vi "UHR-Fleezers Control (host) - 10.7.vi"() -> ()   [LabVIEW 2011] (continued)
        n2234 = Build Array (concatenate)(w3488, w3486) -> (w3487:dbl[])
        n2235 = local read "Scan steps (MCL)"() -> (w3468:u64)
        n2236 = Select(t=w3581, s=w3485, f=w3563) -> (s? t:f=w3567:dbl[])
        n2237 = feedback-in #17(w3567) -> ()
        n2238 = Select(t=w3486, s=w3485, f=w3487) -> (s? t:f=w3469:dbl[])
        n2239 = feedback-in #18(w3469) -> ()
        n2240 = local read "Scan lines (y)"() -> (w3454:u64)
        n2241 = local read "N APD Samp/step"() -> (w3470:dbl)
        n2242 = feedback #19(w3512) -> (w3569:dbl[])
        n2243 = Build Array (concatenate)(w3569, w3512) -> (w3560:dbl[])
        n2244 = feedback #20(w3519) -> (w3579:dbl[])
        n2245 = Build Array (concatenate)(w3579, w3519) -> (w3578:dbl[])
        n2246 = feedback #21(w3514) -> (w3571:dbl[])
        n2247 = Build Array (concatenate)(w3571, w3514) -> (w3572:dbl[])
        n2248 = Select(t=w3512, s=w3485, f=w3560) -> (s? t:f=w3516:dbl[])
        n2249 = feedback-in #19(w3516) -> ()
        n2250 = Select(t=w3519, s=w3485, f=w3578) -> (s? t:f=w3518:dbl[])
        n2251 = feedback-in #20(w3518) -> ()
        n2252 = Select(t=w3514, s=w3485, f=w3572) -> (s? t:f=w3517:dbl[])
        n2253 = feedback-in #21(w3517) -> ()
        n2254 = Multiply(x=w3468, y=u64 2) -> (x*y=w3453:u64)
        n2255 = call "integrate 1D array interval - double.vi"("Ave N"=w3470, "Array In"=w3469) -> ("Array Out"=w3481:dbl[])  [unwired: 1 out]
        n2256 = call "integrate 1D array interval - double.vi"("Ave N"=w3470, "Array In"=w3567) -> ("Array Out"=w3566:dbl[])  [unwired: 1 out]
        n2257 = Array Size(array=w3481) -> (size(s)=w3482:i32)
        n2258 = Array Size(array=w3566) -> (size(s)=w3568:i32)
        n2259 = Multiply(x=w3454, y=w3453) -> (x*y=w3484:u64)
        n2260 = Multiply(x=w3454, y=w3453) -> (x*y=w3576:u64)
        n2261 = call <vilib>:"Mean.vi"("X"=w3516) -> ("mean"=w3500:dbl)  [unwired: 1 out]
        n2262 = Subtract(x=w3484, y=w3482) -> (x-y=w3475:u64)
        n2263 = call <vilib>:"Mean.vi"("X"=w3518) -> ("mean"=w3505:dbl)  [unwired: 1 out]
        n2264 = call <vilib>:"Mean.vi"("X"=w3517) -> ("mean"=w3503:dbl)  [unwired: 1 out]
        n2265 = call <vilib>:"Mean.vi"("X"=w3481) -> ("mean"=w3472:dbl)  [unwired: 1 out]
        n2266 = Subtract(x=w3576, y=w3568) -> (x-y=w3510:u64)
        n2267 = call <vilib>:"Mean.vi"("X"=w3566) -> ("mean"=w3507:dbl)  [unwired: 1 out]
        n2268 = Initialize Array(1.0 ("element"), w3475) -> (w3471:dbl[])
        n2269 = Initialize Array(1.0 ("element"), w3510) -> (w3501:dbl[])
        n2270 = Multiply(x=w3471, y=w3472) -> (x*y=w3473:dbl[])
        n2271 = Multiply(x=w3501, y=w3503) -> (x*y=w3504:dbl[])
        n2272 = Multiply(x=w3501, y=w3505) -> (x*y=w3506:dbl[])
        n2273 = Multiply(x=w3501, y=w3500) -> (x*y=w3502:dbl[])
        n2274 = Multiply(x=w3501, y=w3507) -> (x*y=w3508:dbl[])
        n2275 = Build Array (concatenate)(w3516, w3502) -> (w3570:dbl[])
        n2276 = Build Array (concatenate)(w3518, w3506) -> (w3574:dbl[])
        n2277 = Build Array (concatenate)(w3517, w3504) -> (w3573:dbl[])
        n2278 = Build Array (concatenate)(w3481, w3473) -> (w3483:dbl[])
        n2279 = Build Array (concatenate)(w3566, w3508) -> (w3575:dbl[])
        n2280 = Reshape Array(w3570, w3454, w3453) -> (w3536:dbl[][])
        n2281 = Reshape Array(w3483, w3454, w3453) -> (w3479:dbl[][])
        n2282 = Reshape Array(w3574, w3454, w3453) -> (w3528:dbl[][])
        n2283 = Reshape Array(w3573, w3454, w3453) -> (w3543:dbl[][])
        n2284 = Reshape Array(w3575, w3454, w3453) -> (w3553:dbl[][])
        n2285 = Array Subset(array=w3543, index (col)=0 ("index"), length (col)=w3468) -> (w3548:dbl[][])  [unwired: 2 in]
        n2286 = Array Subset(array=w3543, index (col)=w3468) -> (w3546:dbl[][])  [unwired: 3 in]
        n2287 = Array Subset(array=w3528, index (col)=0 ("index"), length (col)=w3468) -> (w3534:dbl[][])  [unwired: 2 in]
        n2288 = Array Subset(array=w3528, index (col)=w3468) -> (w3532:dbl[][])  [unwired: 3 in]
        n2289 = Array Subset(array=w3479, index (col)=0 ("index"), length (col)=w3468) -> (w3478:dbl[][])  [unwired: 2 in]
        n2290 = Array Subset(array=w3479, index (col)=w3468) -> (w3476:dbl[][])  [unwired: 3 in]
        n2291 = Array Subset(array=w3553, index (col)=0 ("index"), length (col)=w3468) -> (w3552:dbl[][])  [unwired: 2 in]
        n2292 = Array Subset(array=w3553, index (col)=w3468) -> (w3550:dbl[][])  [unwired: 3 in]
        n2293 = Array Subset(array=w3536, index (col)=0 ("index"), length (col)=w3468) -> (w3541:dbl[][])  [unwired: 2 in]
        n2294 = Array Subset(array=w3536, index (col)=w3468) -> (w3539:dbl[][])  [unwired: 3 in]
        n2295 = for {
          tunnel: w3548 -> [w3590] mode=indexing
          tunnel: [w3589] -> w3547 mode=indexing
          workers-P: _ -> [_]
          n2296 = Reverse 1D Array(array=w3590) -> (reversed array=w3589:dbl[])
        }
        n2297 = for {
          tunnel: w3534 -> [w3586] mode=indexing
          tunnel: [w3585] -> w3533 mode=indexing
          workers-P: _ -> [_]
          n2298 = Reverse 1D Array(array=w3586) -> (reversed array=w3585:dbl[])
        }
        n2299 = for {
          tunnel: w3478 -> [w3584] mode=indexing
          tunnel: [w3583] -> w3477 mode=indexing
          workers-P: _ -> [_]
          n2300 = Reverse 1D Array(array=w3584) -> (reversed array=w3583:dbl[])
        }
        n2301 = for {
          tunnel: w3552 -> [w3592] mode=indexing
          tunnel: [w3591] -> w3551 mode=indexing
          workers-P: _ -> [_]
          n2302 = Reverse 1D Array(array=w3592) -> (reversed array=w3591:dbl[])
        }
        n2303 = for {
          tunnel: w3541 -> [w3588] mode=indexing
          tunnel: [w3587] -> w3540 mode=indexing
          workers-P: _ -> [_]
          n2304 = Reverse 1D Array(array=w3588) -> (reversed array=w3587:dbl[])
        }
        n2305 = Index Array(array=w3553, index (row)=0) -> (element=→"Waveform Graph":dbl[])  [unwired: 1 in]
        n2306 = Add(x=w3547, y=w3546) -> (x+y=w3545:dbl[][])
        n2307 = Add(x=w3533, y=w3532) -> (x+y=w3531:dbl[][])
        n2308 = Add(x=w3477, y=w3476) -> (x+y=w3461:dbl[][])
        n2309 = Add(x=w3551, y=w3550) -> (x+y=w3525:dbl[][])
        n2310 = Add(x=w3540, y=w3539) -> (x+y=w3538:dbl[][])
        n2311 = Divide(x=w3531, y=2) -> (x/y=w3529:dbl[][])
        n2312 = Divide(x=w3545, y=2) -> (x/y=w3490:dbl[][])
        n2313 = Divide(x=w3538, y=2) -> (x/y=w3492:dbl[][])
        n2314 = To Single Precision Float(number=w3525) -> (single precision float=w3524:sgl[][])
        n2315 = Transpose 2D Array(2D array=w3529) -> (transposed array=→"Data map":dbl[][])
        n2316 = To Single Precision Float(number=w3461) -> (single precision float=w3465:sgl[][])
        n2317 = To Single Precision Float(number=w3490) -> (single precision float=w3496:sgl[][])
        n2318 = To Single Precision Float(number=w3492) -> (single precision float=w3493:sgl[][])
        n2319 = call "IMAQ ArrayToImage"("Image Pixels (Float)"=w3524, "Image"=w3458) -> ("Image Out"=w3527:T2)  [unwired: 8 in, 1 out]
        n2320 = call "IMAQ ArrayToImage"("Image Pixels (Float)"=w3465, "Image"=w3457) -> ("Image Out"=w3467:T2)  [unwired: 8 in, 1 out]
        n2321 = call "IMAQ ArrayToImage"("Image Pixels (Float)"=w3496, "Image"=w3456) -> ("Image Out"=w3498:T2)  [unwired: 8 in, 1 out]
        n2322 = call "IMAQ ArrayToImage"("Image Pixels (Float)"=w3493, "Image"=w3455) -> ("Image Out"=w3495:T2)  [unwired: 8 in, 1 out]
        n2323 = call "IMAQ Symmetry"("Type of Symmetry"=w3526, "Image Src"=w3527) -> ("Image Dst Out"=w3522:T2)  [unwired: 3 in, 1 out]
        n2324 = call "IMAQ Symmetry"("Type of Symmetry"=w3466, "Image Src"=w3467) -> ("Image Dst Out"=w3463:T2)  [unwired: 3 in, 1 out]
        n2325 = call "IMAQ Symmetry"("Type of Symmetry"=w3497, "Image Src"=w3498) -> ("Image Dst Out"=→"Detection Laser X":T2)  [unwired: 3 in, 1 out]
        n2326 = call "IMAQ Symmetry"("Type of Symmetry"=w3494, "Image Src"=w3495) -> ("Image Dst Out"=→"Detection Laser Y":T2)  [unwired: 3 in, 1 out]
        n2327 = call "IMAQ Set Simple Calibration"("Calibration Axis Info"=T35 {"Origin Pixel"={"X"=0.0, "Y"=0.0}, "Angle Relative to Horizontal (deg)"=0.0, "Axis Reference"=0}, "Grid Descriptor"=T36 {"X Step"=0.3, "Y Step"=0.3, "Unit"=enum."Undefined"}, "Image"=w3522) -> ("Calibrated Image"=→"APD 1":T2)  [unwired: 7 in, 1 out]
        n2328 = call "IMAQ Set Simple Calibration"("Calibration Axis Info"=T35 {"Origin Pixel"={"X"=0.0, "Y"=0.0}, "Angle Relative to Horizontal (deg)"=0.0, "Axis Reference"=0}, "Grid Descriptor"=T36 {"X Step"=0.3, "Y Step"=0.3, "Unit"=enum."Undefined"}, "Image"=w3463) -> ("Calibrated Image"=→"APD 2":T2)  [unwired: 7 in, 1 out]
      }
    }
    n2329 = Subtract(x=w2967, y="APD 2 Offset") -> (x-y=w2964:waveform(dbl))
    n2330 = Subtract(x=w2969, y="APD 1 Offset") -> (x-y=w2965:waveform(dbl))
    n2331 = Index Array(array=w2984, index=3) -> (element=w3044:waveform(dbl))
    n2332 = Index Array(array=w2984, index=6) -> (element=w3041:waveform(dbl))
    n2333 = Build Array(w2965, w2964) -> (→"APD Chart":waveform(dbl)[])
    n2334 = Array Size(array=w3035) -> (size(s)=w3088:i32)
    n2335 = call <vilib>:"Std Deviation and Variance.vi"("X"=w2977) -> ("standard deviation"=w2976:dbl)  [unwired: 1 in, 2 out]
    n2336 = Add Array Elements(numeric array=w2977) -> (sum=w2979:u32)
    n2337 = Add Array Elements(numeric array=w3035) -> (sum=w3098:u32)
    n2338 = call <vilib>:"Std Deviation and Variance.vi"("X"=w3035) -> ("standard deviation"=w3034:dbl)  [unwired: 1 in, 2 out]
    n2339 = Divide(x="T1 offset_x (mV)", y=1000.0) -> (x/y=w3045:dbl)
    n2340 = Divide(x=w2976, y=w2975) -> (x/y=w2972:dbl)
    "Rate sigma (Hz) 2" <- w2972
    n2341 = Multiply(x=w2975, y=w3088) -> (x*y=w2978:dbl)
    "Int. Time (s)" <- w2978
    n2342 = Divide(x=w2979, y=w2978) -> (x/y=w2973:dbl)
    "APD 2 Rate (Hz)" <- w2973
    n2343 = Divide(x=w3098, y=w2978) -> (x/y=w3032:dbl)
    "APD 1 Rate (Hz)" <- w3032
    n2344 = Divide(x=w3034, y=w2975) -> (x/y=w3033:dbl)
    "Rate sigma (Hz)" <- w3033
    n2345 = Divide(x=w2972, y=w2973) -> (x/y=→"Sigma/Mean 2":dbl)
    n2346 = Divide(x=w3033, y=w3032) -> (x/y=→"Sigma/Mean":dbl)
    n2347 = feedback-in #22("Calibration") -> ()
    n2348 = feedback #22(u16 1 ("Calibration")) -> (w3065:u16)
    n2349 = Divide(x="T2 offset_x (mV)", y=1000.0) -> (x/y=w3043:dbl)
    n2350 = case shown="0, Default" "Calibration" {
      tunnel: "T1 alpha_x (nm/V)" -> [_ w3421 w3442]
      tunnel: "T1 kappa_x (pN/nm)" -> [_ _ w3432]
      tunnel: "T2 alpha_x (nm/V)" -> [_ w3420 w3440]
      tunnel: "T2 kappa_x (pN/nm)" -> [_ _ w3433]
      tunnel: w3044 -> [w3403 w3418 w3438]
      tunnel: w3041 -> [w3402 w3416 w3436]
      tunnel: [w3403 w3415 w3435] -> w3074
      tunnel: [w3402 w3414 w3434] -> w3073
      tunnel: ["T1 X (V)" ("Label.Text") "T1 X (nm)" ("Label.Text") "T1 X (pN)" ("Label.Text")] -> w3062
      tunnel: ["T2 X (V)" ("Label.Text") "T2 X (nm)" ("Label.Text") "T2 X (pN)" ("Label.Text")] -> w3061
      tunnel: ["Position (V)" ("Label.Text") "Position (nm)" ("Label.Text") "Force (pN)" ("Label.Text")] -> w3063
      tunnel: w3043 -> [_ w3406 w3425]
      tunnel: w3045 -> [_ w3409 w3427]
      tunnel: ["Mean (V)" ("Label.Text") "Mean (nm)" ("Label.Text") "Mean (pN)" ("Label.Text")] -> w3058
      tunnel: ["Difference (V)" ("Label.Text") "Difference (nm)" ("Label.Text") "Difference (pN)" ("Label.Text")] -> w2992
      frame 0, Default {
      }
      frame 1 {
        n2351 = Unbundle By Name(w3418) -> ("Y"=w3422:dbl[])
        n2352 = Unbundle By Name(w3416) -> ("Y"=w3407:dbl[])
        n2353 = Subtract(x=w3422, y=w3409) -> (x-y=w3410:dbl[])
        n2354 = Subtract(x=w3407, y=w3406) -> (x-y=w3408:dbl[])
        n2355 = Multiply(x=w3408, y=w3420) -> (x*y=w3417:dbl[])
        n2356 = Multiply(x=w3421, y=w3410) -> (x*y=w3419:dbl[])
        n2357 = Bundle By Name(cluster=w3416, "Y"=w3417) -> (w3414:waveform(dbl))
        n2358 = Bundle By Name(cluster=w3418, "Y"=w3419) -> (w3415:waveform(dbl))
      }
      frame 2 {
        n2359 = Unbundle By Name(w3438) -> ("Y"=w3443:dbl[])
        n2360 = Unbundle By Name(w3436) -> ("Y"=w3441:dbl[])
        n2361 = Subtract(x=w3441, y=w3425) -> (x-y=w3426:dbl[])
        n2362 = Subtract(x=w3443, y=w3427) -> (x-y=w3428:dbl[])
        n2363 = Compound Arithmetic op=MULTIPLY(w3426, w3440, w3433) -> (w3437:dbl[])
        n2364 = Compound Arithmetic op=MULTIPLY(w3432, w3442, w3428) -> (w3439:dbl[])
        n2365 = Bundle By Name(cluster=w3436, "Y"=w3437) -> (w3434:waveform(dbl))
        n2366 = Bundle By Name(cluster=w3438, "Y"=w3439) -> (w3435:waveform(dbl))
      }
    }
    n2367 = Not Equal?(x=w3065, y="Calibration") -> (x != y?=w3022:bool)
    n2368 = case shown="True" w3022 {
      tunnel: w3063 -> [_ w3396]
      tunnel: w3062 -> [_ w3395]
      tunnel: w3061 -> [_ w3394]
      tunnel: w3058 -> [_ w3393]
      tunnel: w2992 -> [_ w3392]
      frame False {
      }
      frame True {
        n2369 = property on="Force" class="WFChart (strict)"("YScale.NameLbl.Text"=w3396) -> ()  [unwired: 2 in, 2 out]
        n2370 = property on="T2 X" class="DigNum (strict)"("Caption.Text"=w3394) -> ()  [unwired: 2 in, 2 out]
        n2371 = property on="T1 X" class="DigNum (strict)"("Caption.Text"=w3395) -> ()  [unwired: 2 in, 2 out]
        n2372 = property on="Mean" class="DigNum (strict)"("Caption.Text"=w3393) -> ()  [unwired: 2 in, 2 out]
        n2373 = property on="Difference" class="DigNum (strict)"("Caption.Text"=w3392) -> ()  [unwired: 2 in, 2 out]
      }
    }
    n2374 = Unbundle By Name(w3044) -> ("Y"=w3047:dbl[])
    n2375 = Unbundle By Name(w3041) -> ("Y"=w3050:dbl[])
    n2376 = Subtract(x=w3047, y=w3045) -> (x-y=w3048:dbl[])
    n2377 = Subtract(x=w3050, y=w3043) -> (x-y=w3049:dbl[])
    n2378 = Multiply(x=w3049, y="T2 alpha_x (nm/V)") -> (x*y=w2833:dbl[])
    n2379 = Multiply(x="T1 alpha_x (nm/V)", y=w3048) -> (x*y=w2834:dbl[])
    n2380 = Not(x="Trap Trig. Fl.") -> (.not. x?=w2871:bool)
    n2381 = Multiply(x=w3073, y=-1.0) -> (x*y=w3052:waveform(dbl))
    n2382 = Subtract(x=w2834, y=w2833) -> (x-y=w3040:dbl[])
    n2383 = Unbundle By Name(w3073) -> ("Y"=w3011:dbl[])
    n2384 = Unbundle By Name(w3074) -> ("Y"=w2835:dbl[])
    n2385 = Negate(x=w3040) -> (-x=w2831:dbl[])
    n2386 = Build Array(w3074, w3052) -> (→"Force":waveform(dbl)[])
    n2387 = Subtract(x=w2831, y="Offset (nm)") -> (x-y=w3009:dbl[])
    n2388 = case shown="True" "Read Lateness and Rel Phase" {
      tunnel: w2851 -> [w3369 w3391]
      tunnel: w2850 -> [w3370 w3390]
      tunnel: [w3369 w3389] -> w3038
      tunnel: [w3370 w3388] -> w3037
      frame False {
      }
      frame True {
        n2389 = xnode "Read/Write Control"("FPGA VI Reference In"=w3391, "error in"=w3390) -> ("FPGA VI Reference Out"=w3389:T19, "error out"=w3388:errorcluster, "GI Relative phase"=→"GI relative phase":i16, "Relative phase"=→"Relative phase (AI1)":i16, "AI Late Counter"=→"Late Counter (AI1)":u16, "GI Late Counter"=→"GI Late Counter":u16, "MCL Late Counter"=→"MCL Late Counter":u16, "MCL Relative Phase"=→"Relative Phase (MCL)":i16, "APD Acq Relative Phase"=→"APD Acq Relative Phase":i16, "APD 1 Gate Relative Phase"=→"APD 1 Gate Relative Phase":i16, "APD 2 Gate Relative Phase"=→"APD 2 Gate Relative Phase":i16, "APD Acq Late Counter"=→"APD Acq Late Counter":u16, "APD 1 Gate Late Counter"=→"APD 1 Gate Late Counter":u16, "APD 2 Gate Late Counter"=→"APD 2 Gate Late Counter":u16, "Green FB Relative Phase"=→"Relative phase (Green FB)":i16, "GI Relative phase 2"=→"GI relative phase 2":i16, "GI Late Counter 2"=→"GI Late Counter 2":u16, "Trap Pos FIFO Timeout"=→"Trap Pos FIFO Timeout":u16, "Trap AI FIFO Timeout"=→"Trap AI FIFO Timeout":u16)
      }
    }
    n2390 = call <vilib>:"Mean.vi"("X"=w3011) -> ("mean"=w2837:dbl)  [unwired: 1 out]
    "T2 X" <- w2837
    n2391 = Negate(x=w3011) -> (-x=w3012:dbl[])
    n2392 = call <vilib>:"Mean.vi"("X"=w2835) -> ("mean"=w2838:dbl)  [unwired: 1 out]
    "T1 X" <- w2838
    n2393 = Negate(x=w2837) -> (-x=w2836:dbl)
    n2394 = Bundle By Name(cluster=w3044, "Y"=w3009) -> (w2983:waveform(dbl))
    "Bead Separation" <- w2983
    n2395 = Add(x=w2835, y=w3012) -> (x+y=w3013:dbl[])
    n2396 = Add(x=w2838, y=w2836) -> (x+y=w3060:dbl)
    n2397 = Subtract(x=w2838, y=w2836) -> (x-y=→"Difference":dbl)
    n2398 = Divide(x=w3013, y=2.0) -> (x/y=→"Vec Mean of T1 T2":dbl[])
    n2399 = Divide(x=w3060, y=2.0) -> (x/y=w3015:dbl)
    "Mean" <- w3015
    n2400 = feedback-in #23("Trap Trig. Fl.") -> ()
    n2401 = feedback #23("Trap Trig. Fl.") -> (w2869:bool)
    n2402 = And(x=w2871, y=w2869) -> (x .and. y?=w2870:bool)
    n2403 = case "If have just turned off triggering" shown="True" w2870 {
      tunnel: w2851 -> [_ w3204]
      tunnel: w2850 -> [_ w3203]
      frame False {
      }
      frame True {
        w3202 = FALSE ("FPGA Trap Trig")
        n2404 = xnode "Read/Write Control"("FPGA VI Reference In"=w3204, "error in"=w3203, "FPGA Trap Trig"=w3202) -> ("FPGA VI Reference Out"=w3201:T19, "error out"=w3200:errorcluster)
        n2405 = xnode "Read/Write Control"("FPGA VI Reference In"=w3201, "error in"=w3200, "TTrig?"=w3202) -> ()  [unwired: 2 out]
        n2406 = local write "Initializing"(FALSE ("Initializing")) -> ()
        n2407 = local write "Triggered"(FALSE ("Triggered")) -> ()
        n2408 = local write "Waiting"(FALSE ("Waiting")) -> ()
      }
    }
    n2409 = Not(x=w2869) -> (.not. x?=w2882:bool)
    n2410 = And(x="Trap Trig. Fl.", y=w2882) -> (x .and. y?=w2879:bool)
    n2411 = local read "Tether"() -> (w3016:bool)
    n2412 = Or(x=w2879, y="Reinitialize") -> (x .or. y?=w2865:bool)
    n2413 = feedback #24(w2875) -> (w2880:string)
    n2414 = Select(t=w2875, s=w2879, f=w2880) -> (s? t:f=w2874:string)
    n2415 = Select(t=w2875, s="Reinitialize", f=w2874) -> (s? t:f=w2873:string)
    n2416 = feedback #25(0) -> (w2877:i32)
    n2417 = feedback #26(w3009) -> (w3008:dbl[])
    n2418 = Build Array (concatenate)(w3009, w3008) -> (w2832:dbl[])
    n2419 = case "For determining if there is a tether still" shown="True" w3016 {
      tunnel: w3015 -> [_ w3328]
      frame False {
      }
      frame True {
        n2420 = Greater?(x="Lost Tether Alarm Threshold (pN)", y=w3328) -> (0:w3326:bool)
        n2421 = case shown="True" w3326 {
          frame False {
          }
          frame True {
            w3329 = FALSE ("Value (Signaling)")
            n2422 = flat-sequence {
              frame #0 {
                # "stop only if saving"
                n2423 = local read "Saving..."() -> (w3341:bool)
                n2424 = And(x=w3341, y="TA Cancel Save?") -> (x .and. y?=w3340:bool)
                n2425 = local write "Stop Saving"(w3340) -> ()
              }
              frame #1 {
                n2426 = case shown="True" "TA Green Off?" {
                  frame False {
                  }
                  frame True {
                    w3344 = FALSE ("Fl. Triggered...")
                    n2427 = local write "Fl. Triggered..."(w3344) -> ()
                    n2428 = property on="Green Laser ON/Interlacing" class="Bool (strict)"("Val(Sgnl)"=w3344) -> ()  [unwired: 2 in, 2 out]
                  }
                }
              }
            }
            n2429 = local read "Time tether formed"() -> (w3335:timestamp)
            n2430 = Get Date/Time In Seconds() -> (seconds since 1Jan1904=w3336:timestamp)
            n2431 = Subtract(x=w3336, y=w3335) -> (x-y=w3334:dbl)
            n2432 = Number To Decimal String(number=w3334) -> (decimal integer string=w3331:string)  [unwired: 1 out]
            n2433 = local read "Messages"() -> (w3338:string)
            n2434 = call <vilib>:"Beep.vi"() -> ()  [unwired: 3 in, 9 out]
            n2435 = Concatenate Strings("Lost tether (" ("Message to add"), w3331, " s)." ("string")) -> (w3333:string)
            n2436 = local write "Tether"(FALSE ("Tether")) -> ()
            n2437 = call "Update messages.vi"("Message to add"=w3333, "Old message string"=w3338) -> ("New message string"=w3337:string)
            n2438 = local write "Messages"(w3337) -> ()
            n2439 = local write "Dip for Protein"(w3329) -> ()
            n2440 = property on="Trap Pos. FB ON" class="Bool (strict)"("Val(Sgnl)"=w3329) -> ()  [unwired: 2 in, 2 out]
            n2441 = property on="Trap Trig. Fl." class="Bool (strict)"("Val(Sgnl)"=w3329) -> ()  [unwired: 2 in, 2 out]
          }
        }
      }
    }
    n2442 = case "For triggering actions based on the trap position (e.g., turning the excitation laser on if trap under feedback moves so far)" shown="True" "Trap Trig. Fl." {
      tunnel: w2860 -> [_ w3217]
      tunnel: w2873 -> [_ w3216]
      tunnel: ["" ("t") w3215] -> w2881
      tunnel: w2865 -> [_ w3214]
      tunnel: [0 ("t") w3213] -> w2878
      tunnel: w2877 -> [_ w3212]
      tunnel: w2851 -> [_ w3211]
      tunnel: w2850 -> [_ w3210]
      frame False {
      }
      frame True {
        n2443 = case shown="\"Wait for trigger\"" w3216 {
          tunnel: w3217 -> [w3234 _ _ w3282]
          tunnel: [w3231 w3263 "" ("t") w3285] -> w3215
          tunnel: w3214 -> [_ _ _ w3273]
          tunnel: [w3230 w3260 0 ("t") w3274] -> w3213
          tunnel: w3212 -> [_ w3262 _ w3280]
          tunnel: w3211 -> [w3219 w3257 _ w3276]
          tunnel: w3210 -> [w3218 w3256 _ w3275]
          frame "Wait for trigger" {
            n2444 = local read "Trap Trig. (FPGA)"() -> (w3222:bool)
            n2445 = Subtract(x=w3234, y="Mean T1 Position\nto compare (nm)") -> (x-y=w3227:dbl[])
            n2446 = call <vilib>:"Std Deviation and Variance.vi"("X"=w3227) -> ("mean"=→"mean":dbl, "standard deviation"=→"standard\ndeviation":dbl)  [unwired: 1 in, 1 out]
            n2447 = Array Max & Min(array=w3227) -> (max value=→"max value":dbl, min value=→"min value":dbl)  [unwired: 2 out]
            n2448 = Greater?(x=w3227, y="Threshold (nm)") -> (0:w3237:bool[])
            n2449 = case shown="True" w3222 {
              tunnel: w3219 -> [_ w3243]
              tunnel: w3218 -> [_ w3242]
              tunnel: [FALSE ("TTrig?") w3241] -> w3225
              frame False {
              }
              frame True {
                n2450 = xnode "Read/Write Control"("FPGA VI Reference In"=w3243, "error in"=w3242) -> ("TTrig?"=w3241:bool)  [unwired: 2 out]
              }
            }
            n2451 = Or Array Elements(Boolean array=w3237) -> (logical OR=w3224:bool)
            n2452 = Select(t=w3225, s=w3222, f=w3224) -> (s? t:f=w3223:bool)
            n2453 = Not(x=w3222) -> (.not. x?=w3221:bool)
            n2454 = And(x=w3223, y=w3221) -> (x .and. y?=w3220:bool)
            n2455 = Select(t="Triggered", s=w3223, f="Wait for trigger") -> (s? t:f=w3231:string)
            n2456 = case shown="True" w3223 {
              tunnel: [0 0] -> w3230
              tunnel: w3219 -> [_ w3248]
              tunnel: w3218 -> [_ w3247]
              frame False {
                "Waiting" <- TRUE ("Waiting")
              }
              frame True {
                n2457 = xnode "Read/Write Control"("FPGA VI Reference In"=w3248, "error in"=w3247, "TTrig?"=FALSE) -> ()  [unwired: 2 out]
                n2458 = local read "Messages"() -> (w3251:string)
                n2459 = call <vilib>:"Beep.vi"() -> ()  [unwired: 12 in]
                n2460 = call "Update messages.vi"("Message to add"="Unwinding trigger.", "Old message string"=w3251) -> ("New message string"=w3252:string)
                n2461 = local write "Messages"(w3252) -> ()
                n2462 = local write "Waiting"(FALSE ("Waiting")) -> ()
                "Triggered" <- TRUE ("Triggered")
              }
            }
            n2463 = case "Only need to turn on laser if host triggered" shown="True" w3220 {
              frame False {
              }
              frame True {
                n2464 = property on="Green Laser ON/Interlacing" class="Bool (strict)"("Val(Sgnl)"=TRUE ("Value (Signaling)")) -> ()  [unwired: 2 in, 2 out]
              }
            }
          }
          frame "Triggered" {
            n2465 = local read "Trap Trig. (FPGA)"() -> (w3259:bool)
            n2466 = Increment(x=w3262) -> (x+1=w3260:i32)
            n2467 = Greater Or Equal?(x=w3260, y="Fl. ON time (n)") -> (x >= y?=w3258:bool)
            n2468 = Select(t="Wait for trigger", s=w3258, f="Triggered" ("t")) -> (s? t:f=w3263:string)
            n2469 = And(x=w3258, y=w3259) -> (x .and. y?=w3255:bool)
            n2470 = case shown="True" w3255 {
              tunnel: w3257 -> [_ w3267]
              tunnel: w3256 -> [_ w3266]
              frame False {
              }
              frame True {
                n2471 = xnode "Read/Write Control"("FPGA VI Reference In"=w3267, "error in"=w3266, "FPGA Trap Trig"=TRUE) -> ()  [unwired: 2 out]
              }
            }
            n2472 = case shown="True" w3258 {
              frame False {
              }
              frame True {
                w3269 = FALSE ("Value (Signaling)")
                n2473 = local write "Triggered"(w3269) -> ()
                n2474 = local write "Waiting"(TRUE ("Waiting")) -> ()
                n2475 = property on="Green Laser ON/Interlacing" class="Bool (strict)"("Val(Sgnl)"=w3269) -> ()  [unwired: 2 in, 2 out]
              }
            }
          }
          frame "Do nothing" {
          }
          frame "Initialize", Default {
            n2476 = Increment(x=w3280) -> (x+1=w3284:i32)
            n2477 = Select(t=1, s=w3273, f=w3284) -> (s? t:f=w3274:i32)
            n2478 = feedback #27(w3282) -> (w3288:dbl[])
            n2479 = Build Array (concatenate)(w3282, w3288) -> (w3281:dbl[])
            n2480 = Greater Or Equal?(x=w3274, y="Wait to get offset (n)") -> (x >= y?=w3277:bool)
            n2481 = Select(t=w3282, s=w3273, f=w3281) -> (s? t:f=w3283:dbl[])
            n2482 = feedback-in #27(w3283) -> ()
            n2483 = call <vilib>:"Mean.vi"("X"=w3283) -> ("mean"=w3278:dbl)  [unwired: 1 out]
            n2484 = local write "Mean T1 Position\nto compare (nm)"(w3278) -> ()
            n2485 = case shown="True" w3273 {
              tunnel: w3276 -> [_ w3294]
              tunnel: w3275 -> [_ w3293]
              frame False {
              }
              frame True {
                w3290 = FALSE ("FPGA Trap Trig")
                n2486 = xnode "Read/Write Control"("FPGA VI Reference In"=w3294, "error in"=w3293, "FPGA Trap Trig"=w3290) -> ("FPGA VI Reference Out"=w3292:T19, "error out"=w3291:errorcluster)
                n2487 = xnode "Read/Write Control"("FPGA VI Reference In"=w3292, "error in"=w3291, "TTrig?"=w3290) -> ()  [unwired: 2 out]
              }
            }
            n2488 = Select(t="Wait for trigger", s=w3277, f="Initialize") -> (s? t:f=w3285:string)
            n2489 = case shown="True" w3277 {
              tunnel: w3278 -> [_ w3297]
              tunnel: w3276 -> [_ w3306]
              tunnel: w3275 -> [_ w3305]
              frame False {
                n2490 = local write "Waiting"(FALSE ("Waiting")) -> ()
                "Initializing" <- TRUE ("Initializing")
              }
              frame True {
                n2491 = local read "Threshold (nm)"() -> (w3309:dbl)
                n2492 = local read "AOM X Cal (nm/MHz)"() -> (w3308:dbl)
                n2493 = Add(x=w3297, y=w3309) -> (x+y=w3310:dbl)
                n2494 = Divide(x=w3310, y=w3308) -> (x/y=w3307:dbl)
                n2495 = call "IR AOM freq to word.vi"("Frequency In (MHz)"=w3307) -> ("Frequency Word Out (double)"=w3304:dbl)
                n2496 = local write "Initializing"(FALSE ("Initializing")) -> ()
                n2497 = local write "Waiting"(TRUE ("Waiting")) -> ()
                n2498 = To Quad Integer(1:w3304) -> (0:w3303:i64)
                n2499 = xnode "Read/Write Control"("FPGA VI Reference In"=w3306, "error in"=w3305, "FPGA TTrig Thresh"=w3303) -> ("FPGA VI Reference Out"=w3300:T19, "error out"=w3299:errorcluster)
                n2500 = xnode "Read/Write Control"("FPGA VI Reference In"=w3300, "error in"=w3299, "FPGA Trap Trig"=TRUE) -> ()  [unwired: 2 out]
              }
            }
          }
        }
      }
    }
    n2501 = feedback-in #24(w2881) -> ()
    n2502 = feedback-in #25(w2878) -> ()
    n2503 = Split 1D Array(array=w2832, index=w2895) -> (first subarray=w3005:dbl[])  [unwired: 1 out]
    n2504 = feedback-in #26(w3005) -> ()
    n2505 = call <vilib>:"Mean.vi"("X"=w3005) -> ("mean"=w3004:dbl)  [unwired: 1 out]
    "Bead Mean (nm)" <- w3004
    n2506 = Subtract(x=w3005, y=w3004) -> (x-y=w3003:dbl[])
    n2507 = Square(x=w3003) -> (x^2=w3002:dbl[])
    n2508 = call <vilib>:"Mean.vi"("X"=w3002) -> ("mean"=w3001:dbl)  [unwired: 1 out]
    n2509 = Square Root(x=w3001) -> (sqrt(x)=w3000:dbl)
    n2510 = Multiply(x=10.0, y=w3000) -> (x*y=→"RMS (Ang)":dbl)
    n2511 = xnode "Read/Write Control"("FPGA VI Reference In"=w3038, "error in"=w3037) -> ("FPGA VI Reference Out"=w2863:T19, "error out"=w2862:errorcluster, "AI2 Y Sum Set 1"=w3144:i16, "AI2 Y Sum Set 2"=w3143:i16, "AI1 X Set 1"=w2927:fxp<+/-,16,1>, "AI1 X Set 2"=w2926:fxp<+/-,16,1>, "Trap Pos FB Int Signal"=→"Trap Pos FB Int Signal":fxp<+/-,24,9>, "Trap Pos FB Int-Norm Signal"=→"Trap Pos FB Int-Norm Signal":fxp<+/-,16,1>, "Trap Pos FB Action"=w2920:i64, "Scanning"=→"AOD Scanning":bool, "Scan I"=→"AOD Scan I":u64, "Scanning MCL"=w3146:bool, "Scan I (MCL)"=→"MCL Scan I":u64, "Green FB Signals"=w3083:T46, "TTrig Sig"=w2849:i64, "TTrig Fin Thresh"=w2845:i64)
    "MCL Scanning" <- w3146
    "Trap Pos FB Action" <- w2920
    n2512 = local read "FB Trig Integrate"() -> (w2843:u32)
    n2513 = Divide(x=w2849, y=w2843) -> (x/y=w2842:dbl)
    "TTrig Sig (Int)" <- w2842
    n2514 = Divide(x=w2845, y=w2843) -> (x/y=w2840:dbl)
    "TTrig Fin Thresh (Int)" <- w2840
    n2515 = local read "AOM X Cal (nm/MHz)"() -> (w2848:dbl)
    n2516 = local read "AI2 (V)"() -> (w3145:cluster{"Set 1":dbl, "Set 2":dbl})
    n2517 = Bundle By Name(cluster=w3145, "Set 1"=w3144, "Set 2"=w3143) -> (w3141:cluster{"Set 1":dbl, "Set 2":dbl})
    n2518 = Divide(x=w2920, y=327.67) -> (x/y=→"Action (%)":dbl)
    n2519 = local read "Trap X (AI1)"() -> (w2940:T10)
    n2520 = call "IR AOM word double to freq.vi"("Frequency Word In (double)"=w2840) -> ("Frequency Out (MHz)"=w2839:dbl)
    n2521 = call "IR AOM word double to freq.vi"("Frequency Word In (double)"=w2842) -> ("Frequency Out (MHz)"=w2841:dbl)
    n2522 = Divide(x=w3141, y=3276.7) -> (x/y=w3140:cluster{"Set 1":dbl, "Set 2":dbl})
    n2523 = Multiply(x=w2841, y=w2848) -> (x*y=w2847:dbl)
    "TTrig Sig (nm)" <- w2847
    n2524 = Multiply(x=w2839, y=w2848) -> (x*y=w2846:dbl)
    "TTrig Fin Thresh (nm)" <- w2846
    n2525 = local write "AI2 (V)"(w3140) -> ()
    n2526 = Bundle(cluster=w2940, "Trap 1"=w2927, "Trap 2"=w2926) -> (→"Trap X (AI1)":T10)
    n2527 = Bundle(w2847, w2846) -> (→"TTrig":cluster{dbl, dbl})  [unwired: 1 in]
    n2528 = Divide(x=w3083, y=3276.7) -> (x/y=w3079:T47)
    n2529 = Unbundle By Name(w3079) -> ("Green FB Ch 0"=w3082:dbl, "Green FB Ch 1"=w3081:dbl, "Green FB Ch 2"=w3080:dbl)
    n2530 = Divide(x=w3082, y=w3080) -> (x/y=w3078:dbl)
    n2531 = Divide(x=w3081, y=w3080) -> (x/y=w3077:dbl)
    n2532 = flat-sequence "To save data" {
      tunnel: [w4165] -> w3164
      tunnel: [w4166] -> w3163
      tunnel: w3114 -> [w4159]
      tunnel: w2868 -> [w4163]
      tunnel: ["Save Calibration"] -> w3137
      tunnel: w3134 -> [w4162]
      tunnel: [w4155] -> w3133
      tunnel: [w4152] -> w3132
      tunnel: [w4149] -> w3131
      tunnel: w3113 -> [w4151]
      tunnel: w3020 -> [w4145]
      tunnel: [w4145] -> w3019
      tunnel: ["Start Saving"] -> w2985
      tunnel: [w4139] -> w2908
      tunnel: [w4138] -> w2907
      tunnel: w3164 -> [w4400]
      tunnel: w3163 -> [w4399]
      tunnel: w2909 -> [w4398]
      tunnel: w3137 -> [w4397]
      tunnel: w3133 -> [w4395]
      tunnel: w3132 -> [w4394]
      tunnel: w3131 -> [w4393]
      tunnel: w2994 -> [w4392]
      tunnel: w3030 -> [w4391]
      tunnel: w3019 -> [w4390]
      tunnel: w2985 -> [w4389]
      tunnel: w2983 -> [w4388]
      tunnel: w2959 -> [w4387]
      tunnel: w2908 -> [w4386]
      tunnel: w2907 -> [w4385]
      tunnel: w2906 -> [w4384]
      frame #0 {
        n2533 = Or(x="Save N Sets", y="Start Saving") -> (x .or. y?=w4146:bool)
        n2534 = To Double Precision Float(number=w4162) -> (double precision float=w4156:dbl)
        n2535 = Build Array(w4146, "Save Calibration", w4159, w4151) -> (w4161:bool[])
        n2536 = Compound Arithmetic op=OR("Save Calibration", w4159, w4146, w4151) -> (w4164:bool)
        n2537 = Boolean Array To Number(Boolean array=w4161) -> (number=w4158:u32)
        n2538 = feedback #28(FALSE ("Save APD Data\nwith Trap Data")) -> (w4140:bool)
        n2539 = feedback #29(refnum<k0> refnum) -> (w4167:refnum<file>)
        n2540 = feedback #30(refnum<k0> refnum) -> (w4142:refnum<file>)
        n2541 = feedback #31(FALSE ("Save APD Data\nwith Trap Data")) -> (w4150:bool)
        n2542 = feedback #32(refnum<k0> refnum) -> (w4153:refnum<file>)
        n2543 = feedback #33(0) -> (w4169:i32)
        n2544 = feedback #34() -> (w4157:u32)  [unwired: 1 out]
        n2545 = case shown="True" w4164 {
          tunnel: [w4176 1] -> w4165
          tunnel: w4169 -> [w4178 _]
          tunnel: [w4177 w4196] -> w4166
          tunnel: w4167 -> [w4177 _]
          tunnel: w4163 -> [_ w4216]
          tunnel: w4156 -> [_ w4214]
          tunnel: w4158 -> [_ w4217]
          tunnel: [w4175 w4195] -> w4155
          tunnel: w4157 -> [w4175 _]
          tunnel: [w4174 w4193] -> w4152
          tunnel: w4153 -> [w4174 _]
          tunnel: [w4173 w4192] -> w4149
          tunnel: w4150 -> [w4173 _]
          tunnel: "Start Saving" -> [_ w4190]
          tunnel: w4145 -> [_ w4189]
          tunnel: [w4172 w4180] -> w4138
          tunnel: w4142 -> [w4172 _]
          tunnel: [w4171 w4179] -> w4139
          tunnel: w4140 -> [w4171 _]
          frame False {
            n2546 = Increment(x=w4178) -> (x+1=w4176:i32)
          }
          frame True {
            w4186 = FALSE ("Start Saving")
            w4191 = 9.0  # File Version
            w4199 = FALSE ("prepend array or string size? (T)")
            w4197 = T24."big-endian, network order" ("byte order (0:big-endian, network order)")
            n2547 = local read "BD 1 Frequency 1 (MHz)"() -> (w4213:dbl)
            n2548 = local read "BD 2 Frequency 1 (MHz)"() -> (w4212:dbl)
            n2549 = local read "BD 1 Frequency 2 (MHz)"() -> (w4211:dbl)
            n2550 = local read "BD 2 Frequency 2 (MHz)"() -> (w4210:dbl)
            n2551 = local read "BD 1 Frequency 3 (MHz)"() -> (w4209:dbl)
            n2552 = local read "BD 2 Frequency 3 (MHz)"() -> (w4208:dbl)
            n2553 = Array Size(array=w4189) -> (size(s)=w4188:i32)
            n2554 = To Double Precision Float(number=w4188) -> (double precision float=w4187:dbl)
            n2555 = local write "Save Calibration"(w4186) -> ()
            n2556 = local write "Start Saving"(w4186) -> ()
            n2557 = Build Array("Save APD Data\nwith Trap Data", "Save Trap Pos. Data") -> (w4183:bool[])
            n2558 = Boolean Array To Number(Boolean array=w4183) -> (number=w4182:u32)
            n2559 = Build Array(w4213, w4212, w4211, w4210, w4209, w4208) -> (w4207:dbl[])
            n2560 = case shown="4" w4217 {
              tunnel: w4216 -> [w4288 w4308 w4324 w4362]
              tunnel: w4187 -> [w4293 w4315 w4344 w4381]
              tunnel: w4214 -> [w4292 w4314 w4343 w4380]
              tunnel: [w4289 w4310 w4335 w4372] -> w4205
              tunnel: [w4280 "Cal sets to save" w4325 w4363] -> w4195
              tunnel: w4207 -> [w4290 w4311 w4337 w4374]
              tunnel: "Save APD Data\nwith Trap Data" -> [w4287 _ w4321 w4360]
              tunnel: [w4287 w4302 w4321 w4360] -> w4192
              tunnel: w4191 -> [w4283 w4303 w4319 w4358]
              tunnel: w4190 -> [w4282 _ _ _]
              tunnel: [w4273 w4302 w4318 w4348] -> w4179
              tunnel: "Save Trap Pos. Data" -> [w4273 _ w4318 w4348]
              tunnel: w4182 -> [w4272 _ w4317 w4347]
              frame 1, Default {
                # "timeseries"
                n2561 = case shown="True" "Profile" {
                  tunnel: [w4296 w4300] -> w4277
                  tunnel: [w4296 w4299] -> w4276
                  tunnel: [w4296 w4298] -> w4275
                  tunnel: [w4296 w4297] -> w4274
                  frame False {
                    w4296 = 0.0 ("f")
                  }
                  frame True {
                    n2562 = local read "Current Position"() -> (w4301:cluster{dbl, dbl, dbl})
                    n2563 = local read "Y change (mm)"() -> (w4297:dbl)
                    n2564 = Unbundle(w4301) -> (w4300:dbl, w4299:dbl, w4298:dbl)
                  }
                }
                n2565 = local read "Save ave N"() -> (w4295:dbl)
                n2566 = Multiply(x=w4295, y=w4288) -> (x*y=w4294:dbl)
                n2567 = To Double Precision Float(number=w4272) -> (double precision float=w4286:dbl)
                n2568 = Build Array(w4283, w4288, w4294, w4293, w4292, 0.0 ("f")) -> (w4291:dbl[])
                n2569 = Build Array(w4286, w4277, w4276, w4275, w4274) -> (w4284:dbl[])
                n2570 = Select(t=u32 4000000000, s=w4282, f="N sets to save") -> (s? t:f=w4280:u32)
                n2571 = Build Array (concatenate)(w4291, w4290, w4284) -> (w4289:dbl[])
              }
              frame 2 {
                w4305 = 0.0 ("f")
                w4302 = FALSE ("Save APD Data\nwith Trap Data")
                # "calibration"
                n2572 = Boolean To (0,1)(Boolean=w4302) -> (0, 1=w4307:i16)
                n2573 = To Double Precision Float(number=w4307) -> (double precision float=w4306:dbl)
                n2574 = Build Array(w4306, w4305, w4305, w4305, w4305) -> (w4304:dbl[])
                n2575 = Build Array(w4303, w4308, w4308, w4315, w4314, 1.0 ("t")) -> (w4312:dbl[])
                n2576 = Build Array (concatenate)(w4312, w4311, w4304) -> (w4310:dbl[])
                "Calibrating Trap..." <- TRUE ("Calibrating...")
              }
              frame 4 {
                w4322 = 0.0 ("f")
                # "scan dir (x/y = 0/1)"
                # "cycles/step"
                # "n scans (f/b)"
                # "steps"
                # "freq. range"
                # "AOD raster scan"
                n2577 = local read "Number of F/B Scans (AOD)"() -> (w4329:u16)
                n2578 = local read "Cycles/step (AOD)"() -> (w4331:u64)
                n2579 = local read "Scan Range (MHz)"() -> (w4334:dbl)
                n2580 = local read "Scan steps (AOD)"() -> (w4333:u64)
                n2581 = local read "Scan BD"() -> (w4341:bool)
                n2582 = local read "Save ave N"() -> (w4346:dbl)
                n2583 = Boolean To (0,1)(Boolean=w4341) -> (0, 1=w4340:i16)
                n2584 = To Double Precision Float(number=w4329) -> (double precision float=w4328:dbl)
                n2585 = To Double Precision Float(number=w4333) -> (double precision float=w4332:dbl)
                n2586 = To Double Precision Float(number=w4331) -> (double precision float=w4330:dbl)
                n2587 = To Double Precision Float(number=w4340) -> (double precision float=w4339:dbl)
                n2588 = Multiply(x=w4346, y=w4324) -> (x*y=w4345:dbl)
                n2589 = To Double Precision Float(number=w4317) -> (double precision float=w4323:dbl)
                n2590 = Build Array(w4323, w4322, w4322, w4322, w4322) -> (w4320:dbl[])
                n2591 = local read "N sets should be saved"() -> (w4326:dbl)
                n2592 = Build Array(w4339, w4334, w4332, w4330, w4328) -> (w4336:dbl[])
                n2593 = Build Array(w4319, w4324, w4345, w4344, w4343, 2.0 ("t")) -> (w4338:dbl[])
                n2594 = Round Toward +Infinity(x=w4326) -> (ceil(x): smallest int >= x=w4327:dbl)
                n2595 = Build Array (concatenate)(w4338, w4337, w4320, w4336) -> (w4335:dbl[])
                n2596 = To Unsigned Long Integer(number=w4327) -> (unsigned 32bit integer=w4325:u32)
              }
              frame 8 {
                w4355 = 0.0 ("f")
                # "MCL raster scan"
                n2597 = local read "Number of scans (MCL)"() -> (w4350:u64)
                n2598 = local read "Scan lines (y)"() -> (w4349:u64)
                n2599 = local read "2D or 1D Scan"() -> (w4352:bool)
                n2600 = local read "Scan Range (V)\n(of steps)"() -> (w4371:dbl)
                n2601 = local read "Fast Scan Dir"() -> (w4378:bool)
                n2602 = local read "Cycles/step (MCL)"() -> (w4368:u64)
                n2603 = local read "Scan steps (MCL)"() -> (w4370:u64)
                n2604 = Select(t=w4349, s=w4352, f=w4350) -> (s? t:f=w4351:u64)
                n2605 = Boolean To (0,1)(Boolean=w4352) -> (0, 1=w4354:i16)
                n2606 = local read "Save ave N"() -> (w4383:dbl)
                n2607 = local read "Initial X"() -> (w4357:dbl)
                n2608 = local read "Initial Y"() -> (w4356:dbl)
                n2609 = To Double Precision Float(number=w4354) -> (double precision float=w4353:dbl)
                n2610 = Boolean To (0,1)(Boolean=w4378) -> (0, 1=w4377:i16)
                n2611 = To Double Precision Float(number=w4351) -> (double precision float=w4366:dbl)
                n2612 = To Double Precision Float(number=w4370) -> (double precision float=w4369:dbl)
                n2613 = To Double Precision Float(number=w4368) -> (double precision float=w4367:dbl)
                n2614 = To Double Precision Float(number=w4377) -> (double precision float=w4376:dbl)
                n2615 = Multiply(x=w4383, y=w4362) -> (x*y=w4382:dbl)
                n2616 = To Double Precision Float(number=w4347) -> (double precision float=w4361:dbl)
                n2617 = local read "N sets should be saved (MCL)"() -> (w4364:dbl)
                n2618 = Build Array(w4361, w4353, w4355, w4355, w4355) -> (w4359:dbl[])
                n2619 = Build Array(w4376, w4371, w4369, w4367, w4366, w4357, w4356) -> (w4373:dbl[])
                n2620 = Build Array(w4358, w4362, w4382, w4381, w4380, 3.0 ("t")) -> (w4375:dbl[])
                n2621 = Round Toward +Infinity(x=w4364) -> (ceil(x): smallest int >= x=w4365:dbl)
                n2622 = Build Array (concatenate)(w4375, w4374, w4359, w4373) -> (w4372:dbl[])
                n2623 = To Unsigned Long Integer(number=w4365) -> (unsigned 32bit integer=w4363:u32)
              }
            }
            n2624 = local read "Index"() -> (w4222:dbl)
            n2625 = call "Create new save file.vi"("Insert"="", "Ext"=".dat", "Index In"=w4222) -> ("Path Out"=w4181:path, "Index Out"=w4194:dbl)
            n2626 = local write "Save file name"(w4181) -> ()
            n2627 = local write "Index"(w4194) -> ()
            n2628 = local write "Save index"(w4194) -> ()
            n2629 = Array Size(array=w4205) -> (size(s)=w4206:i32)
            n2630 = Open/Create/Replace File(file path (use dialog)=w4181, operation (0:open)=T25."create", access (0:read/write)=enum16{"read/write", "read-only", "write-only"}."write-only") -> (refnum out=w4219:refnum<file>)  [unwired: 1 in, 4 out]
            n2631 = local write "Saving..."(TRUE ("Saving...")) -> ()
            n2632 = To Double Precision Float(number=w4206) -> (double precision float=w4204:dbl)
            n2633 = String Length(string="Comment (data description)") -> (length=w4202:i32)
            n2634 = To Double Precision Float(number=w4202) -> (double precision float=w4201:dbl)
            n2635 = Deny Access(7:w4219) -> (3:w4218:refnum<file>)  [unwired: 1 in, 2 out]
            n2636 = Build Array (concatenate)(w4204, w4205, w4201) -> (w4203:dbl[])
            n2637 = case "If fluorescence data to be saved" shown="True" w4192 {
              tunnel: w4181 -> [_ w4271]
              tunnel: [refnum<k0> refnum w4251] -> w4193
              frame False {
              }
              frame True {
                w4250 = 0.0
                n2638 = local read "APD Integration Time (s)"() -> (w4256:dbl)
                n2639 = local read "N APD Samp/step"() -> (w4249:dbl)
                n2640 = Path To String(path=w4271) -> (string=w4270:string)
                n2641 = String Length(string=w4270) -> (length=w4269:i32)
                n2642 = Subtract(x=w4269, y=4) -> (x-y=w4267:i32)
                n2643 = String Subset(string=w4270, length (rest)=w4267) -> (substring=w4266:string)  [unwired: 1 out]
                n2644 = Build Array(w4256, w4249, w4250, w4250, w4250, w4250, w4250, w4250) -> (w4253:dbl[])
                n2645 = Concatenate Strings(w4266, "_fl.dat" ("string")) -> (w4264:string)
                n2646 = Array Size(array=w4253) -> (size(s)=w4255:i32)
                n2647 = String To Path(string=w4264) -> (path=w4260:path)
                n2648 = Open/Create/Replace File(file path (use dialog)=w4260, operation (0:open)=T25."create", access (0:read/write)=enum16{"read/write", "read-only", "write-only"}."write-only") -> (refnum out=w4261:refnum<file>)  [unwired: 1 in, 4 out]
                n2649 = Deny Access(7:w4261) -> (3:w4257:refnum<file>)  [unwired: 1 in, 2 out]
                n2650 = To Double Precision Float(number=w4255) -> (double precision float=w4254:dbl)
                n2651 = Build Array (concatenate)(w4254, w4253) -> (w4252:dbl[])
                n2652 = Write to Binary File(file (use dialog)=w4257, data=w4252, 5:FALSE ("prepend array or string size? (T)"), 9:T24."big-endian, network order" ("byte order (0:big-endian, network order)")) -> (refnum out=w4251:refnum<file>)  [unwired: 1 in, 3 out]
              }
            }
            n2653 = case shown="True" w4179 {
              tunnel: w4181 -> [_ w4233]
              tunnel: [refnum<k0> refnum w4232] -> w4180
              frame False {
              }
              frame True {
                w4228 = 0.0 ("element")
                n2654 = Path To String(path=w4233) -> (string=w4247:string)
                n2655 = Build Array(w4228, w4228, w4228, w4228, w4228, w4228, w4228, w4228) -> (w4229:dbl[])
                n2656 = String Length(string=w4247) -> (length=w4246:i32)
                n2657 = Subtract(x=w4246, y=4) -> (x-y=w4244:i32)
                n2658 = Array Size(array=w4229) -> (size(s)=w4231:i32)
                n2659 = String Subset(string=w4247, length (rest)=w4244) -> (substring=w4243:string)  [unwired: 1 out]
                n2660 = To Double Precision Float(number=w4231) -> (double precision float=w4230:dbl)
                n2661 = Concatenate Strings(w4243, "_pos.dat" ("string")) -> (w4241:string)
                n2662 = Build Array (concatenate)(w4230, w4229) -> (w4227:dbl[])
                n2663 = String To Path(string=w4241) -> (path=w4237:path)
                n2664 = Open/Create/Replace File(file path (use dialog)=w4237, operation (0:open)=T25."create", access (0:read/write)=enum16{"read/write", "read-only", "write-only"}."write-only") -> (refnum out=w4238:refnum<file>)  [unwired: 1 in, 4 out]
                n2665 = Deny Access(7:w4238) -> (3:w4234:refnum<file>)  [unwired: 1 in, 2 out]
                n2666 = Write to Binary File(file (use dialog)=w4234, data=w4227, 5:FALSE ("prepend array or string size? (T)"), 9:T24."big-endian, network order" ("byte order (0:big-endian, network order)")) -> (refnum out=w4232:refnum<file>)  [unwired: 1 in, 3 out]
              }
            }
            n2667 = Write to Binary File(file (use dialog)=w4218, data=w4203, 5:w4199, 9:w4197) -> (refnum out=w4200:refnum<file>)  [unwired: 1 in, 3 out]
            n2668 = Write to Binary File(file (use dialog)=w4200, data="Comment (data description)", 5:w4199, 9:w4197) -> (refnum out=w4196:refnum<file>)  [unwired: 1 in, 3 out]
          }
        }
        n2669 = feedback-in #28(w4139) -> ()
        n2670 = feedback-in #29(w4166) -> ()
        n2671 = feedback-in #30(w4138) -> ()
        n2672 = feedback-in #31(w4149) -> ()
        n2673 = feedback-in #32(w4152) -> ()
        n2674 = feedback-in #33(w4165) -> ()
        n2675 = feedback-in #34(w4155) -> ()
      }
      frame #1 {
        n2676 = local read "Saving..."() -> (w4396:bool)
        n2677 = case shown="True" w4396 {
          tunnel: w4400 -> [_ w4410]
          tunnel: w4399 -> [_ w4424]
          tunnel: w4398 -> [_ w4420]
          tunnel: w4397 -> [_ w4419]
          tunnel: w4395 -> [_ w4418]
          tunnel: w4394 -> [_ w4413]
          tunnel: w4393 -> [_ w4412]
          tunnel: w4392 -> [_ w4411]
          tunnel: w4391 -> [_ w4409]
          tunnel: w4390 -> [_ w4407]
          tunnel: w4389 -> [_ w4406]
          tunnel: w4388 -> [_ w4405]
          tunnel: w4387 -> [_ w4404]
          tunnel: w4386 -> [_ w4403]
          tunnel: w4385 -> [_ w4402]
          tunnel: w4384 -> [_ w4401]
          frame False {
          }
          frame True {
            n2678 = Multiply(x=w4410, y=w4409) -> (x*y=→"Time (s)":dbl)
            n2679 = Less Or Equal?(x=w4410, y=w4418) -> (x <= y?=w4422:bool)
            n2680 = Or(x="Stop Saving", y="Abort save 2") -> (x .or. y?=w4414:bool)
            n2681 = Not(x=w4414) -> (.not. x?=w4423:bool)
            n2682 = And(x=w4422, y=w4423) -> (x .and. y?=w4421:bool)
            n2683 = case shown="True" w4421 {
              tunnel: w4424 -> [w4431 w4499]
              tunnel: [0.0 w4502] -> w4417
              tunnel: w4410 -> [_ w4500]
              tunnel: w4418 -> [_ w4501]
              tunnel: w4420 -> [_ w4496]
              tunnel: w4419 -> [_ _]
              tunnel: w4413 -> [w4429 w4489]
              tunnel: w4412 -> [w4428 w4490]
              tunnel: w4411 -> [_ w4488]
              tunnel: w4407 -> [_ w4487]
              tunnel: w4406 -> [_ w4441]
              tunnel: w4405 -> [_ w4480]
              tunnel: w4404 -> [_ w4458]
              tunnel: w4403 -> [w4425 w4439]
              tunnel: w4402 -> [w4426 w4438]
              tunnel: w4401 -> [_ w4435]
              frame False {
                w4427 = FALSE
                n2684 = Close File(refnum=w4431) -> ()  [unwired: 1 in, 2 out]
                n2685 = case shown="True" w4428 {
                  tunnel: w4429 -> [_ w4433]
                  frame False {
                  }
                  frame True {
                    n2686 = Close File(refnum=w4433) -> ()  [unwired: 1 in, 2 out]
                  }
                }
                n2687 = case shown="True" w4425 {
                  tunnel: w4426 -> [_ w4432]
                  frame False {
                  }
                  frame True {
                    n2688 = Close File(refnum=w4432) -> ()  [unwired: 1 in, 2 out]
                  }
                }
                n2689 = local write "Raster Scanning..."(w4427) -> ()
                n2690 = local write "Calibrating Trap..."(w4427) -> ()
                n2691 = call <vilib>:"Beep.vi"() -> ()  [unwired: 3 in, 9 out]
                n2692 = local write "Stop Saving"(w4427) -> ()
                "Saving..." <- w4427
              }
              frame True {
                n2693 = local read "Calibrating Trap..."() -> (w4491:bool)
                n2694 = case "Write fl. data" shown="True" w4490 {
                  tunnel: w4489 -> [_ w4525]
                  tunnel: w4488 -> [_ w4524]
                  frame False {
                  }
                  frame True {
                    n2695 = Write to Binary File(file (use dialog)=w4525, data=w4524, 5:FALSE ("prepend array or string size? (T)"), 9:T24."big-endian, network order" ("byte order (0:big-endian, network order)")) -> ()  [unwired: 1 in, 4 out]
                  }
                }
                n2696 = Greater?(x="Save ave N", y=1.0) -> (0:w4494:bool)
                n2697 = Not(x=w4491) -> (.not. x?=w4493:bool)
                n2698 = And(x=w4493, y=w4494) -> (x .and. y?=w4436:bool)
                n2699 = case shown="True" w4436 {
                  tunnel: w4435 -> [w4505 w4516]
                  tunnel: [w4505 w4508] -> w4434
                  tunnel: "Save ave N" -> [_ w4509]
                  frame False {
                  }
                  frame True {
                    w4506 = 2 ("dimension size")
                    n2700 = Array Size(array=w4516) -> (size(s)=w4510:i32)
                    n2701 = Divide(x=w4510, y=w4506) -> (x/y=w4514:dbl)
                    n2702 = Reshape Array(w4516, w4514, w4506) -> (w4515:u64[][])
                    n2703 = Transpose 2D Array(2D array=w4515) -> (transposed array=w4513:u64[][])
                    n2704 = for {
                      tunnel: w4513 -> [w4518] mode=indexing
                      tunnel: [w4517] -> w4507 mode=indexing
                      tunnel: w4509 -> [w4519]
                      workers-P: _ -> [_]
                      n2705 = call "downsample 1D array - U64.vi"("Ave N"=w4519, "Array In"=w4518) -> ("Array Out"=w4517:u64[])  [unwired: 1 in]
                    }
                    n2706 = Transpose 2D Array(2D array=w4507) -> (transposed array=w4512:u64[][])
                    n2707 = Divide(x=w4510, y=w4509) -> (x/y=w4511:dbl)
                    n2708 = Reshape Array(w4512, w4511) -> (w4508:u64[])
                  }
                }
                n2709 = case shown="False" w4436 {
                  tunnel: w4496 -> [w4528 w4540]
                  tunnel: [w4528 w4532] -> w4492
                  tunnel: "Save ave N" -> [_ w4533]
                  tunnel: w4487 -> [_ w4531]
                  frame False {
                  }
                  frame True {
                    n2710 = Array Size(array=w4540) -> (size(s)=w4534:i32)
                    n2711 = Array Size(array=w4531) -> (size(s)=w4530:i32)
                    n2712 = Divide(x=w4534, y=w4530) -> (x/y=w4538:dbl)
                    n2713 = Reshape Array(w4540, w4538, w4530) -> (w4539:i16[][])
                    n2714 = Transpose 2D Array(2D array=w4539) -> (transposed array=w4537:i16[][])
                    n2715 = for {
                      tunnel: w4537 -> [w4543] mode=indexing
                      tunnel: [w4542] -> w4529 mode=indexing
                      tunnel: w4533 -> [w4541]
                      workers-P: _ -> [_]
                      n2716 = call "downsample 1D array - I16.vi"("Ave N"=w4541, "Array In"=w4543) -> ("Array Out"=w4542:i16[])  [unwired: 1 out]
                    }
                    n2717 = Transpose 2D Array(2D array=w4529) -> (transposed array=w4536:i16[][])
                    n2718 = Divide(x=w4534, y=w4533) -> (x/y=w4535:dbl)
                    n2719 = Reshape Array(w4536, w4535) -> (w4532:i16[])
                  }
                }
                n2720 = Index Array(array=w4458, index=1) -> (element=w4461:waveform(dbl))
                n2721 = Index Array(array=w4458, index=0) -> (element=w4463:waveform(dbl))
                n2722 = Unbundle By Name(w4461) -> ("Y"=w4465:dbl[])
                n2723 = Unbundle By Name(w4463) -> ("Y"=w4473:dbl[])
                n2724 = case "Write trap pos. data" shown="True" w4439 {
                  tunnel: w4438 -> [_ w4521]
                  tunnel: w4434 -> [_ w4520]
                  frame False {
                  }
                  frame True {
                    n2725 = Write to Binary File(file (use dialog)=w4521, data=w4520, 5:FALSE ("prepend array or string size? (T)"), 9:T24."big-endian, network order" ("byte order (0:big-endian, network order)")) -> ()  [unwired: 1 in, 4 out]
                  }
                }
                n2726 = Write to Binary File(file (use dialog)=w4499, data=w4492, 5:FALSE ("prepend array or string size? (T)"), 9:T24."big-endian, network order" ("byte order (0:big-endian, network order)")) -> ()  [unwired: 1 in, 4 out]
                n2727 = feedback #35(w4465) -> (w4467:dbl[])
                n2728 = Build Array (concatenate)(w4467, w4465) -> (w4466:dbl[])
                n2729 = Select(t=w4465, s=w4441, f=w4466) -> (s? t:f=w4451:dbl[])
                n2730 = feedback-in #35(w4451) -> ()
                n2731 = feedback #36(w4473) -> (w4486:dbl[])
                n2732 = Build Array (concatenate)(w4486, w4473) -> (w4485:dbl[])
                n2733 = Select(t=w4473, s=w4441, f=w4485) -> (s? t:f=w4460:dbl[])
                n2734 = feedback-in #36(w4460) -> ()
                n2735 = Divide(x=w4500, y=w4501) -> (x/y=w4503:dbl)
                n2736 = Multiply(x=w4503, y=100.0) -> (x*y=w4502:dbl)
                n2737 = Build Array(w4460, w4451) -> (→"Saved APD":dbl[][])
                n2738 = Array Size(array=w4460) -> (size(s)=w4478:i32)
                n2739 = Unbundle By Name(w4480) -> ("Y"=w4484:dbl[])
                n2740 = Subtract(x=w4478, y="N pts to average") -> (x-y=w4454:i32)
                n2741 = Multiply(x="N pts to average", y=u16 2) -> (x*y=w4455:u16)
                n2742 = Subtract(x=w4478, y=w4455) -> (x-y=w4453:i32)
                n2743 = feedback #37(w4484) -> (w4483:dbl[])
                n2744 = Build Array (concatenate)(w4483, w4484) -> (w4482:dbl[])
                n2745 = Select(t=w4484, s=w4441, f=w4482) -> (s? t:f=w4481:dbl[])
                "Trap Delta Graph" <- w4481
                n2746 = feedback-in #37(w4481) -> ()
                n2747 = Array Subset(array=w4460, index=w4454, length="N pts to average") -> (w4477:dbl[])
                n2748 = Array Subset(array=w4460, index=w4453, length="N pts to average") -> (w4476:dbl[])
                n2749 = Array Subset(array=w4451, index=w4454, length="N pts to average") -> (w4457:dbl[])
                n2750 = Array Subset(array=w4451, index=w4453, length="N pts to average") -> (w4456:dbl[])
                n2751 = call <vilib>:"Mean.vi"("X"=w4477) -> ("mean"=w4475:dbl)  [unwired: 1 out]
                n2752 = call <vilib>:"Mean.vi"("X"=w4457) -> ("mean"=w4450:dbl)  [unwired: 1 out]
                n2753 = call <vilib>:"Mean.vi"("X"=w4476) -> ("mean"=w4474:dbl)  [unwired: 1 out]
